vi "BarLIV_Ex_DataOut.vi"(2 "error in (no error)":errorcluster, 3 "Bar_LIV_Data":path=path "D:/LabVIEW_prog/Trumpf_Database_Connect/All_DM17_TestFiles/Averaging_DM17-128.xlsx") -> (0 "error out":errorcluster, 1 "Output test data":T1={"Test Date"="3/22/2019", "Bar SN"=["30101152", "30101562", "30101566", "30101586", "30101731"], "Bar WO"=["DM17-20", "DM17-20", "DM17-20", "DM17-20", "DM17-20"], "Wafer ID"=["", "", "", "", ""], "Last update"=["31 emitters/Pass", "Pass", "Fail", "Pass", "31 emitters/Pass"], "Current value(A)"=[30.0, 60.0, 90.0, 120.0, 150.0, 180.0, 210.0, 240.0, 270.0, 300.0, 330.0], "Power(W)"=[[0.06, 24.48, 57.61, 91.3, 125.0, 158.3, 191.3, 222.8, 253.6, 282.9, 311.2], [0.18, 25.92, 59.94, 94.3, 128.7, 162.8, 196.5, 229.2, 261.0, 291.7, 320.8], [0.14, 25.11, 58.98, 93.3, 127.7, 161.8, 195.3, 228.2, 260.1, 290.9, 320.2], [0.12, 24.93, 58.6, 92.9, 127.3, 161.3, 194.7, 227.6, 259.4, 290.1, 319.4], [0.18, 24.92, 58.52, 92.7, 126.8, 160.3, 192.9, 224.9, 255.6, 285.6, 313.9]], "Voltage(V)"=[[1.375, 1.414, 1.445, 1.475, 1.504, 1.532, 1.56, 1.587, 1.613, 1.639, 1.664], [1.374, 1.413, 1.443, 1.473, 1.502, 1.53, 1.557, 1.584, 1.61, 1.635, 1.659], [1.375, 1.413, 1.444, 1.473, 1.502, 1.53, 1.558, 1.584, 1.61, 1.635, 1.66], [1.375, 1.415, 1.447, 1.478, 1.507, 1.537, 1.565, 1.593, 1.62, 1.647, 1.673], [1.375, 1.415, 1.446, 1.475, 1.505, 1.533, 1.561, 1.588, 1.614, 1.64, 1.665]], "Centroid(nm)"=[[933.8844535901926, 935.13, 935.9, 936.78, 937.76, 938.84, 939.97, 941.25, 942.63, 944.11, 945.73], [934.4128321548195, 935.59, 936.37, 937.19, 938.12, 939.14, 940.27, 941.5, 942.83, 944.21, 945.83], [934.2026831077322, 935.39, 936.11, 936.93, 937.91, 938.84, 939.97, 941.04, 942.37, 943.75, 945.28], [934.0565390864778, 935.23, 935.95, 936.78, 937.71, 938.68, 939.76, 940.89, 942.12, 943.49, 945.02], [933.6435339561624, 934.87, 935.64, 936.47, 937.45, 938.48, 939.55, 940.73, 942.06, 943.54, 945.12]], "Junction Temp(C)"=[[37.77351299658973, 41.87070513411404, 44.403599870956086, 47.29833671306133, 50.522020923587704, 54.074652502535216, 57.79175776569309, 62.00228408148247, 66.54175776569298, 71.41017881832462, 76.7391261867457], [37.88793822106435, 41.76020086968448, 44.3259903433686, 47.0233587644214, 50.08256929073703, 53.4378324486317, 57.154937711789586, 61.20099034336859, 65.57599034336872, 70.11546402757924, 75.4444113960003], [37.77392541989149, 41.679573091824864, 44.04799414445653, 46.745362565508955, 49.96904677603533, 53.02825730235133, 56.74536256550921, 60.26509940761426, 64.6400994076144, 69.1795730918249, 74.21246782866693], [37.54999732043578, 41.41006611491691, 43.778487167548576, 46.508750325443074, 49.56796085175907, 52.758750325443, 56.3113819043905, 60.02848716754838, 64.0745397991274, 68.58111874649582, 73.61401348333784], [37.885239489759186, 41.91966726554078, 44.45256200238283, 47.1828251602777, 50.40650937080407, 53.794667265540824, 57.314404107645885, 61.19598305501451, 65.57098305501427, 70.43940410764591, 75.63677252869867]], "Efficiency(%)"=[[0.14545454545454548, 28.854314002828858, 44.29834678969627, 51.5819209039548, 55.40780141843972, 57.40498984624311, 58.3943833943834, 58.49611426170973, 58.23058023925972, 57.53508236729713, 56.67249417249417], [0.43668122270742354, 30.573248407643316, 46.153846153846146, 53.34917402127177, 57.12383488681757, 59.11401597676108, 60.09725662904854, 60.290404040404034, 60.041407867494826, 59.46992864424057, 58.59681809048898], [0.3393939393939394, 29.617834394904456, 45.38319482917821, 52.78343516632722, 56.679982245894365, 58.75090777051562, 59.69191270860077, 60.0273569023569, 59.8343685300207, 59.30682976554535, 58.45198977729098], [0.29090909090909095, 29.36395759717314, 44.997312447208785, 52.37934145241317, 56.314974563149754, 58.3026097014386, 59.242355089000455, 59.53128269512451, 59.30498399634201, 58.712811171827575, 57.85288630476914], [0.4363636363636364, 29.35217903415784, 44.96695865990472, 52.37288135593221, 56.16832779623478, 58.092338914256736, 58.845062688752634, 59.01028547439127, 58.653448988021474, 58.04878048780488, 57.12985712985713]]})   [LabVIEW 2017]
uses:
  <vilib>/addons/_office/excel.llb/Excel Get Data ([str]).vi
  <vilib>/addons/_office/excel.llb/Excel Get Data (str).vi
  <vilib>/addons/_office/excel.llb/Excel Get Data ([dbl]).vi
  <vilib>/Utility/NIReport.llb/NI_report.lvclass
  <vilib>/addons/_office/NI_ReportGenerationToolkit.lvlib
  <vilib>/Utility/NIReport.llb/Excel/NI_Excel.lvclass
panel:
  in  "Current Input":dbl[](array[numeric])=[30.0, 60.0, 90.0, 120.0, 150.0, 180.0, 210.0, 240.0, 270.0, 300.0, 330.0]
  out "Current Size":i32=11
  out "Device Number":i32=4
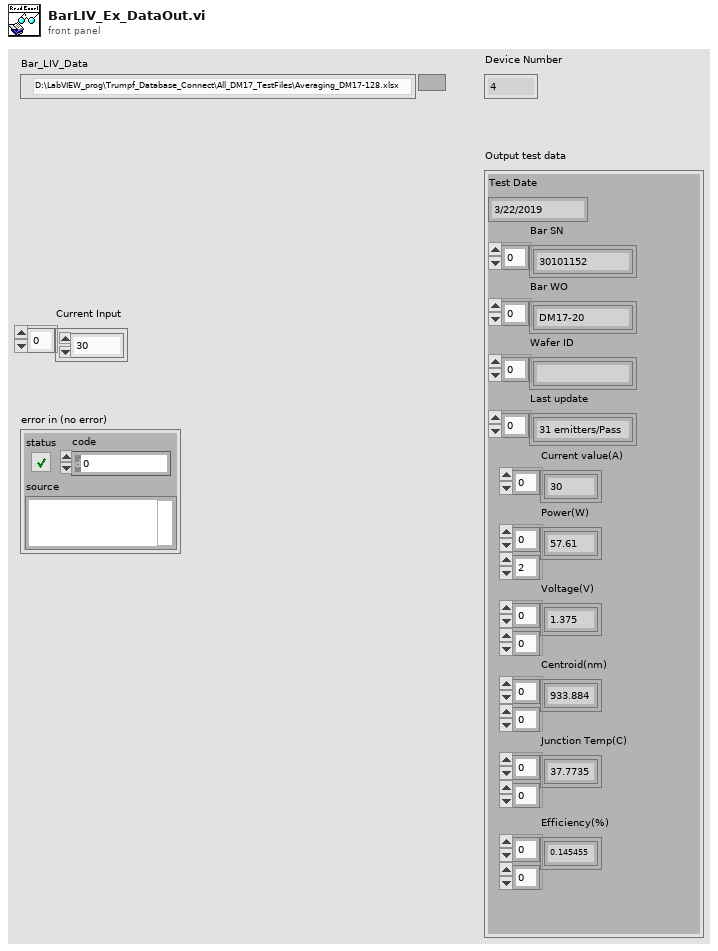
[diagram p1: front panel]
types:
  T1 = cluster{"Test Date":string, "Bar SN":string[], "Bar WO":string[], "Wafer ID":string[], "Last update":string[], "Current value(A)":dbl[], "Power(W)":dbl[][], "Voltage(V)":dbl[][], "Centroid(nm)":dbl[][], "Junction Temp(C)":dbl[][], "Efficiency(%)":dbl[][]}
  T2 = enum16{"Standard Report", "HTML", "Word", "Excel"}
  T3 = cluster{"date/time string":string, "data":string[], "data":string[], "data":string[], "data":string[], "Current Input":dbl[], "data":dbl[][], "data":dbl[][], "data":dbl[][], "data":dbl[][], dbl[][]}
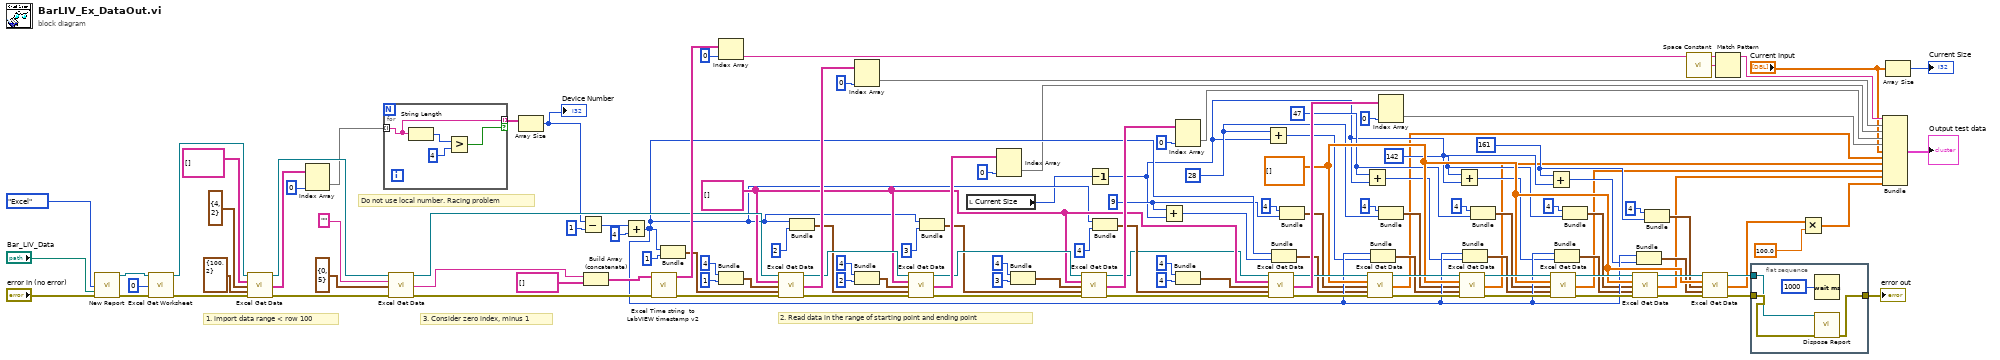
[diagram p0: block diagram]
diagram:
  w34 = 161 ("element")
  w36 = 142 ("element")
  w38 = 47 ("element")
  w40 = 28 ("element")
  w42 = 9 ("element")
  w51 = dbl[][] []
  w71 = string[][] []
  # "Do not use local number. Racing problem"
  # "3. Consider zero index, minus 1"
  # "2. Read data in the range of starting point and ending point"
  # "1. import data range < row 100"
  n1 = call <vilib>:"New Report.vi"("report type"=T2."Excel", "template (empty)"="Bar_LIV_Data", "error in (no error)"="error in (no error)") -> ("report out"=w122:refnum<class "NI_report.lvclass">, "error out"=w121:errorcluster)  [unwired: 11 in]
  n2 = call <vilib>:"Excel Get Worksheet.vi"("report in"=w122, "worksheet index (0)"=0, "error in (no error)"=w121) -> ("report out"=w119:refnum<class "NI_report.lvclass">, "error out"=w116:errorcluster)  [unwired: 11 out]
  n3 = call-poly <vilib>:"Excel Get Data.vi"("report in"=w119, "data type"=string[][] [], "start (-1, -1)"=cluster{"row":i32, "column":i32} {"row"=4, "column"=2}, "end (-1, -1)"=cluster{"row":i32, "column":i32} {"row"=100, "column"=2}, "error in (no error)"=w116) -> ("report out"=w113:refnum<class "NI_report.lvclass">, "data"=w115:string[][], "error out"=w111:errorcluster)  [unwired: 8 in]
  n4 = Index Array(array=w115, index (col)=0 ("disabled index (col)")) -> (element=w3:string[])  [unwired: 1 in]
  n5 = for {
    tunnel: w3 -> [w127] mode=indexing
    tunnel: [w127] -> w2 mode=indexing if=w126
    n6 = String Length(string=w127) -> (length=w129:i32)
    n7 = Greater?(x=w129, y=4) -> (0:w126:bool)
  }
  n8 = call-poly <vilib>:"Excel Get Data.vi"("report in"=w113, "data type"="", "start (0, 0)"=cluster{"start row":i32, "start column":i32} {"start row"=0, "start column"=5}, "error in (no error)"=w111) -> ("report out"=w101:refnum<class "NI_report.lvclass">, "data"=w108:string, "error out"=w102:errorcluster)  [unwired: 9 in]
  n9 = Array Size(array=w2) -> (size(s)=w1:i32)
  "Device Number" <- w1
  n10 = Subtract(x=w1, y=1) -> (x-y=w5:i32)
  n11 = Build Array (concatenate)(w108, string[] []) -> (w107:string[])
  n12 = Add(x=w5, y=4 ("element")) -> (x+y=w43:i32)
  n13 = call "Excel Time string  to LabVIEW timestamp v2.vi"("Error In"=w102, "XLDateIn"=w107) -> ("Error Out"=w94:errorcluster, "DateOut"=w106:string[])  [unwired: 7 in, 1 out]
  n14 = Bundle(w43, "element"=1) -> (w95:cluster{i32, "element":i32})  [unwired: 1 in]
  n15 = Index Array(array=w106, index=0) -> (element=w104:string)
  n16 = Bundle("element"=4, "element"=1) -> (w96:cluster{"element":i32, "element":i32})  [unwired: 1 in]
  n17 = call-poly <vilib>:"Excel Get Data.vi"("report in"=w101, "data type"=w71, "start (-1, -1)"=w96, "end (-1, -1)"=w95, "error in (no error)"=w94) -> ("report out"=w89:refnum<class "NI_report.lvclass">, "data"=w93:string[][], "error out"=w83:errorcluster)  [unwired: 8 in]
  n18 = Bundle(w43, "element"=2) -> (w84:cluster{i32, "element":i32})  [unwired: 1 in]
  n19 = Index Array(array=w93, index (col)=0 ("disabled index (col)")) -> (element=w17:string[])  [unwired: 1 in]
  n20 = Bundle("element"=4, "element"=2) -> (w85:cluster{"element":i32, "element":i32})  [unwired: 1 in]
  n21 = call-poly <vilib>:"Excel Get Data.vi"("report in"=w89, "data type"=w71, "start (-1, -1)"=w85, "end (-1, -1)"=w84, "error in (no error)"=w83) -> ("report out"=w82:refnum<class "NI_report.lvclass">, "data"=w91:string[][], "error out"=w81:errorcluster)  [unwired: 8 in]
  n22 = Bundle(w43, "element"=3) -> (w76:cluster{i32, "element":i32})  [unwired: 1 in]
  n23 = local read "Current Size"() -> (w22:i32)
  n24 = Index Array(array=w91, index (col)=0 ("disabled index (col)")) -> (element=w16:string[])  [unwired: 1 in]
  n25 = Bundle("element"=4, "element"=3) -> (w77:cluster{"element":i32, "element":i32})  [unwired: 1 in]
  n26 = call-poly <vilib>:"Excel Get Data.vi"("report in"=w82, "data type"=w71, "start (-1, -1)"=w77, "end (-1, -1)"=w76, "error in (no error)"=w81) -> ("report out"=w65:refnum<class "NI_report.lvclass">, "data"=w75:string[][], "error out"=w64:errorcluster)  [unwired: 8 in]
  n27 = Decrement(x=w22) -> (x-1=w21:i32)
  n28 = Bundle(w43, "element"=4) -> (w66:cluster{i32, "element":i32})  [unwired: 1 in]
  n29 = Add(x=w42, y=w21) -> (x+y=w41:i32)
  n30 = Index Array(array=w75, index (col)=0 ("disabled index (col)")) -> (element=w15:string[])  [unwired: 1 in]
  n31 = Bundle("element"=4, "element"=4) -> (w67:cluster{"element":i32, "element":i32})  [unwired: 1 in]
  n32 = Add(x=w40, y=w21) -> (x+y=w39:i32)
  n33 = call-poly <vilib>:"Excel Get Data.vi"("report in"=w65, "data type"=w71, "start (-1, -1)"=w67, "end (-1, -1)"=w66, "error in (no error)"=w64) -> ("report out"=w62:refnum<class "NI_report.lvclass">, "data"=w63:string[][], "error out"=w57:errorcluster)  [unwired: 8 in]
  n34 = Bundle(w43, w41) -> (w31:cluster{i32, i32})  [unwired: 1 in]
  n35 = Bundle("element"=4, "element"=w42) -> (w32:cluster{"element":i32, "element":i32})  [unwired: 1 in]
  n36 = Add(x=w38, y=w21) -> (x+y=w37:i32)
  n37 = call-poly <vilib>:"Excel Get Data.vi"("report in"=w62, "data type"=w51, "start (-1, -1)"=w32, "end (-1, -1)"=w31, "error in (no error)"=w57) -> ("report out"=w61:refnum<class "NI_report.lvclass">, "data"=w12:dbl[][], "error out"=w56:errorcluster)  [unwired: 8 in]
  n38 = Bundle(w43, w39) -> (w29:cluster{i32, i32})  [unwired: 1 in]
  n39 = Index Array(array=w63, index (col)=0 ("disabled index (col)")) -> (element=w14:string[])  [unwired: 1 in]
  n40 = Bundle("element"=4, "element"=w40) -> (w30:cluster{"element":i32, "element":i32})  [unwired: 1 in]
  n41 = Add(x=w36, y=w21) -> (x+y=w35:i32)
  n42 = call-poly <vilib>:"Excel Get Data.vi"("report in"=w61, "data type"=w51, "start (-1, -1)"=w30, "end (-1, -1)"=w29, "error in (no error)"=w56) -> ("report out"=w60:refnum<class "NI_report.lvclass">, "data"=w11:dbl[][], "error out"=w55:errorcluster)  [unwired: 8 in]
  n43 = Bundle(w43, w37) -> (w27:cluster{i32, i32})  [unwired: 1 in]
  n44 = Bundle("element"=4, "element"=w38) -> (w28:cluster{"element":i32, "element":i32})  [unwired: 1 in]
  n45 = Add(x=w34, y=w21) -> (x+y=w33:i32)
  n46 = call-poly <vilib>:"Excel Get Data.vi"("report in"=w60, "data type"=w51, "start (-1, -1)"=w28, "end (-1, -1)"=w27, "error in (no error)"=w55) -> ("report out"=w59:refnum<class "NI_report.lvclass">, "data"=w10:dbl[][], "error out"=w54:errorcluster)  [unwired: 8 in]
  n47 = Bundle(w43, w35) -> (w25:cluster{i32, i32})  [unwired: 1 in]
  n48 = Bundle("element"=4, "element"=w36) -> (w26:cluster{"element":i32, "element":i32})  [unwired: 1 in]
  n49 = call-poly <vilib>:"Excel Get Data.vi"("report in"=w59, "data type"=w51, "start (-1, -1)"=w26, "end (-1, -1)"=w25, "error in (no error)"=w54) -> ("report out"=w58:refnum<class "NI_report.lvclass">, "data"=w9:dbl[][], "error out"=w53:errorcluster)  [unwired: 8 in]
  n50 = Bundle(w43, w33) -> (w23:cluster{i32, i32})  [unwired: 1 in]
  n51 = Bundle("element"=4, "element"=w34) -> (w24:cluster{"element":i32, "element":i32})  [unwired: 1 in]
  n52 = call <vilib>:"Space Constant.vi"() -> ("String"=w103:string)
  n53 = call-poly <vilib>:"Excel Get Data.vi"("report in"=w58, "data type"=w51, "start (-1, -1)"=w24, "end (-1, -1)"=w23, "error in (no error)"=w53) -> ("report out"=w49:refnum<class "NI_report.lvclass">, "data"=w19:dbl[][], "error out"=w52:errorcluster)  [unwired: 8 in]
  n54 = Match Pattern(string=w104, regular expression=w103) -> (before substring=w18:string)  [unwired: 1 in, 3 out]
  n55 = flat-sequence {
    tunnel: [w133] -> w73
    tunnel: w52 -> [w132]
    tunnel: w49 -> [w131]
    frame #0 {
      n56 = call-dynamic "Dispose Report.vi"("report in"=w131, "error in (no error)"=w132) -> ("error out"=w133:errorcluster)  [unwired: 13 in]
      n57 = Wait (ms)(milliseconds to wait=u32 1000) -> ()  [unwired: 1 out]
    }
  }
  n58 = Multiply(x=w19, y=100.0) -> (x*y=w8:dbl[][])
  n59 = Bundle("date/time string"=w18, "data"=w17, "data"=w16, "data"=w15, "data"=w14, "Current Input"="Current Input", "data"=w12, "data"=w11, "data"=w10, "data"=w9, w8) -> (→"Output test data":T3)  [unwired: 1 in]
  n60 = Array Size(array="Current Input") -> (size(s)=→"Current Size":i32)
  "error out" <- w73
